vi "um_to_I16_USB7855R.vi"(6 "-10 to 10V?":bool, 7 "Calibration Constant":cluster{"LSB Weight":u32, "Offset":i32}, 8 "Max Value [um]":dbl, 11 "Input":dbl[](array[numeric])=[0.0, 0.0]) -> (2 "Array":i16[](array[numeric]))   [LabVIEW 2023]
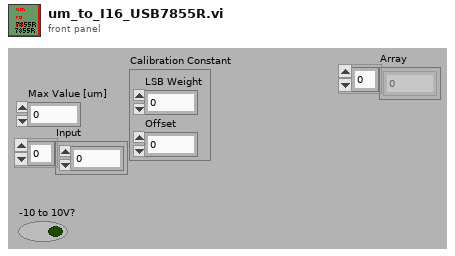
[diagram p1: front panel]
types:
  T1 = enum16{"USB 7855 (AI)", "USB 7855 (AO)", "USB 7855 OEM (AI)", "USB 7855 OEM (AO)", "USB 7856  (AI)", "USB 7856 (AO)", "USB 7856 OEM (AI)", "USB 7856 OEM (AO)"}
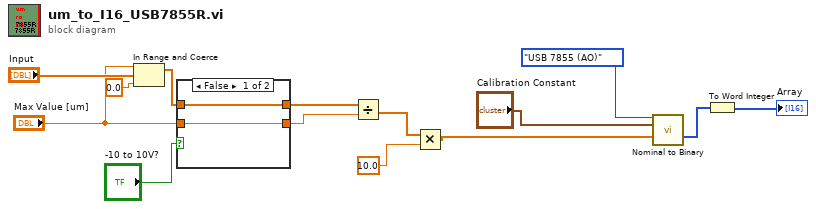
[diagram p0: block diagram]
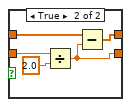
[diagram p2: hidden frame]
diagram:
  n1 = In Range and Coerce(upper limit="Max Value [um]", x="Input", lower limit=0.0 ("n")) -> (coerced(x)=w10:dbl[])  [unwired: 1 out]
  n2 = case shown="False" "-10 to 10V?" {
    tunnel: w10 -> [w16 w19]
    tunnel: [w16 w17] -> w12
    tunnel: [w15 w18] -> w11
    tunnel: "Max Value [um]" -> [w15 w20]
    frame False {
    }
    frame True {
      n3 = Divide(x=w20, y=2.0) -> (x/y=w18:dbl)
      n4 = Subtract(x=w19, y=w18) -> (x-y=w17:dbl[])
    }
  }
  n5 = Divide(x=w12, y=w11) -> (x/y=w7:dbl[])
  n6 = Multiply(x=w7, y=10.0 ("n")) -> (x*y=w3:dbl[])
  n7 = call "Nominal to Binary.vi"("Target Type"=T1."USB 7855 (AO)", "Calibration"="Calibration Constant", "Nominal Value"=w3) -> ("Binary Value"=w2:i32[])  [unwired: 12 in]
  n8 = To Word Integer(number=w2) -> (16bit integer=→"Array":i16[])
